vi "Vision Assistant2.vi"(0 "Image In":T1, 1 "Color Plane (Color Plane Extraction 1)":i32(ring)=2 items=["Red", "Green", "Blue", "Hue", "Saturation", "Luminance", "Value", "Intensity"], 2 "Range (Threshold 1)":cluster{"Lower value":sgl, "Upper value":sgl}={"Lower value"=199.0, "Upper value"=255.0}, 3 "Number of Erosion (Adv. Morphology 1)":i32=1, 4 "Square/Hexa (Square) (Adv. Morphology 1)":bool, 5 "Connectivity 4/8 (8) (Adv. Morphology 1)":bool=TRUE, 6 "Low Pass/High Pass (Low) (Adv. Morphology 1)":bool, 7 "error in":errorcluster) -> (20 "Image Out":T1, 21 "Number of Matches (Shape Matching 1)":i32, 22 "Shape Report (calibrated) (Shape Matching 1)":T2(array[cluster]) {"Score" format="%.2f"; "Centroid"."y" format="%.2f"; "Centroid"."x" format="%.2f"}, 23 "Centroid (Centroid 1)":cluster{"X Centroid":sgl, "Y Centroid":sgl} {"Y Centroid" format="%.2f"; "X Centroid" format="%.2f"}, 24 "Calibrated Centroid (Centroid 1)":cluster{"X Centroid":sgl, "Y Centroid":sgl} {"Y Centroid" format="%.2f"; "X Centroid" format="%.2f"}, 27 "error out":errorcluster)   [LabVIEW 2016]
uses:
  <vilib>/vision/Image Controls.llb/IMAQ Image.ctl
  Camera Global.vi
  <vilib>/vision/NI_Vision_Development_Module.lvlib
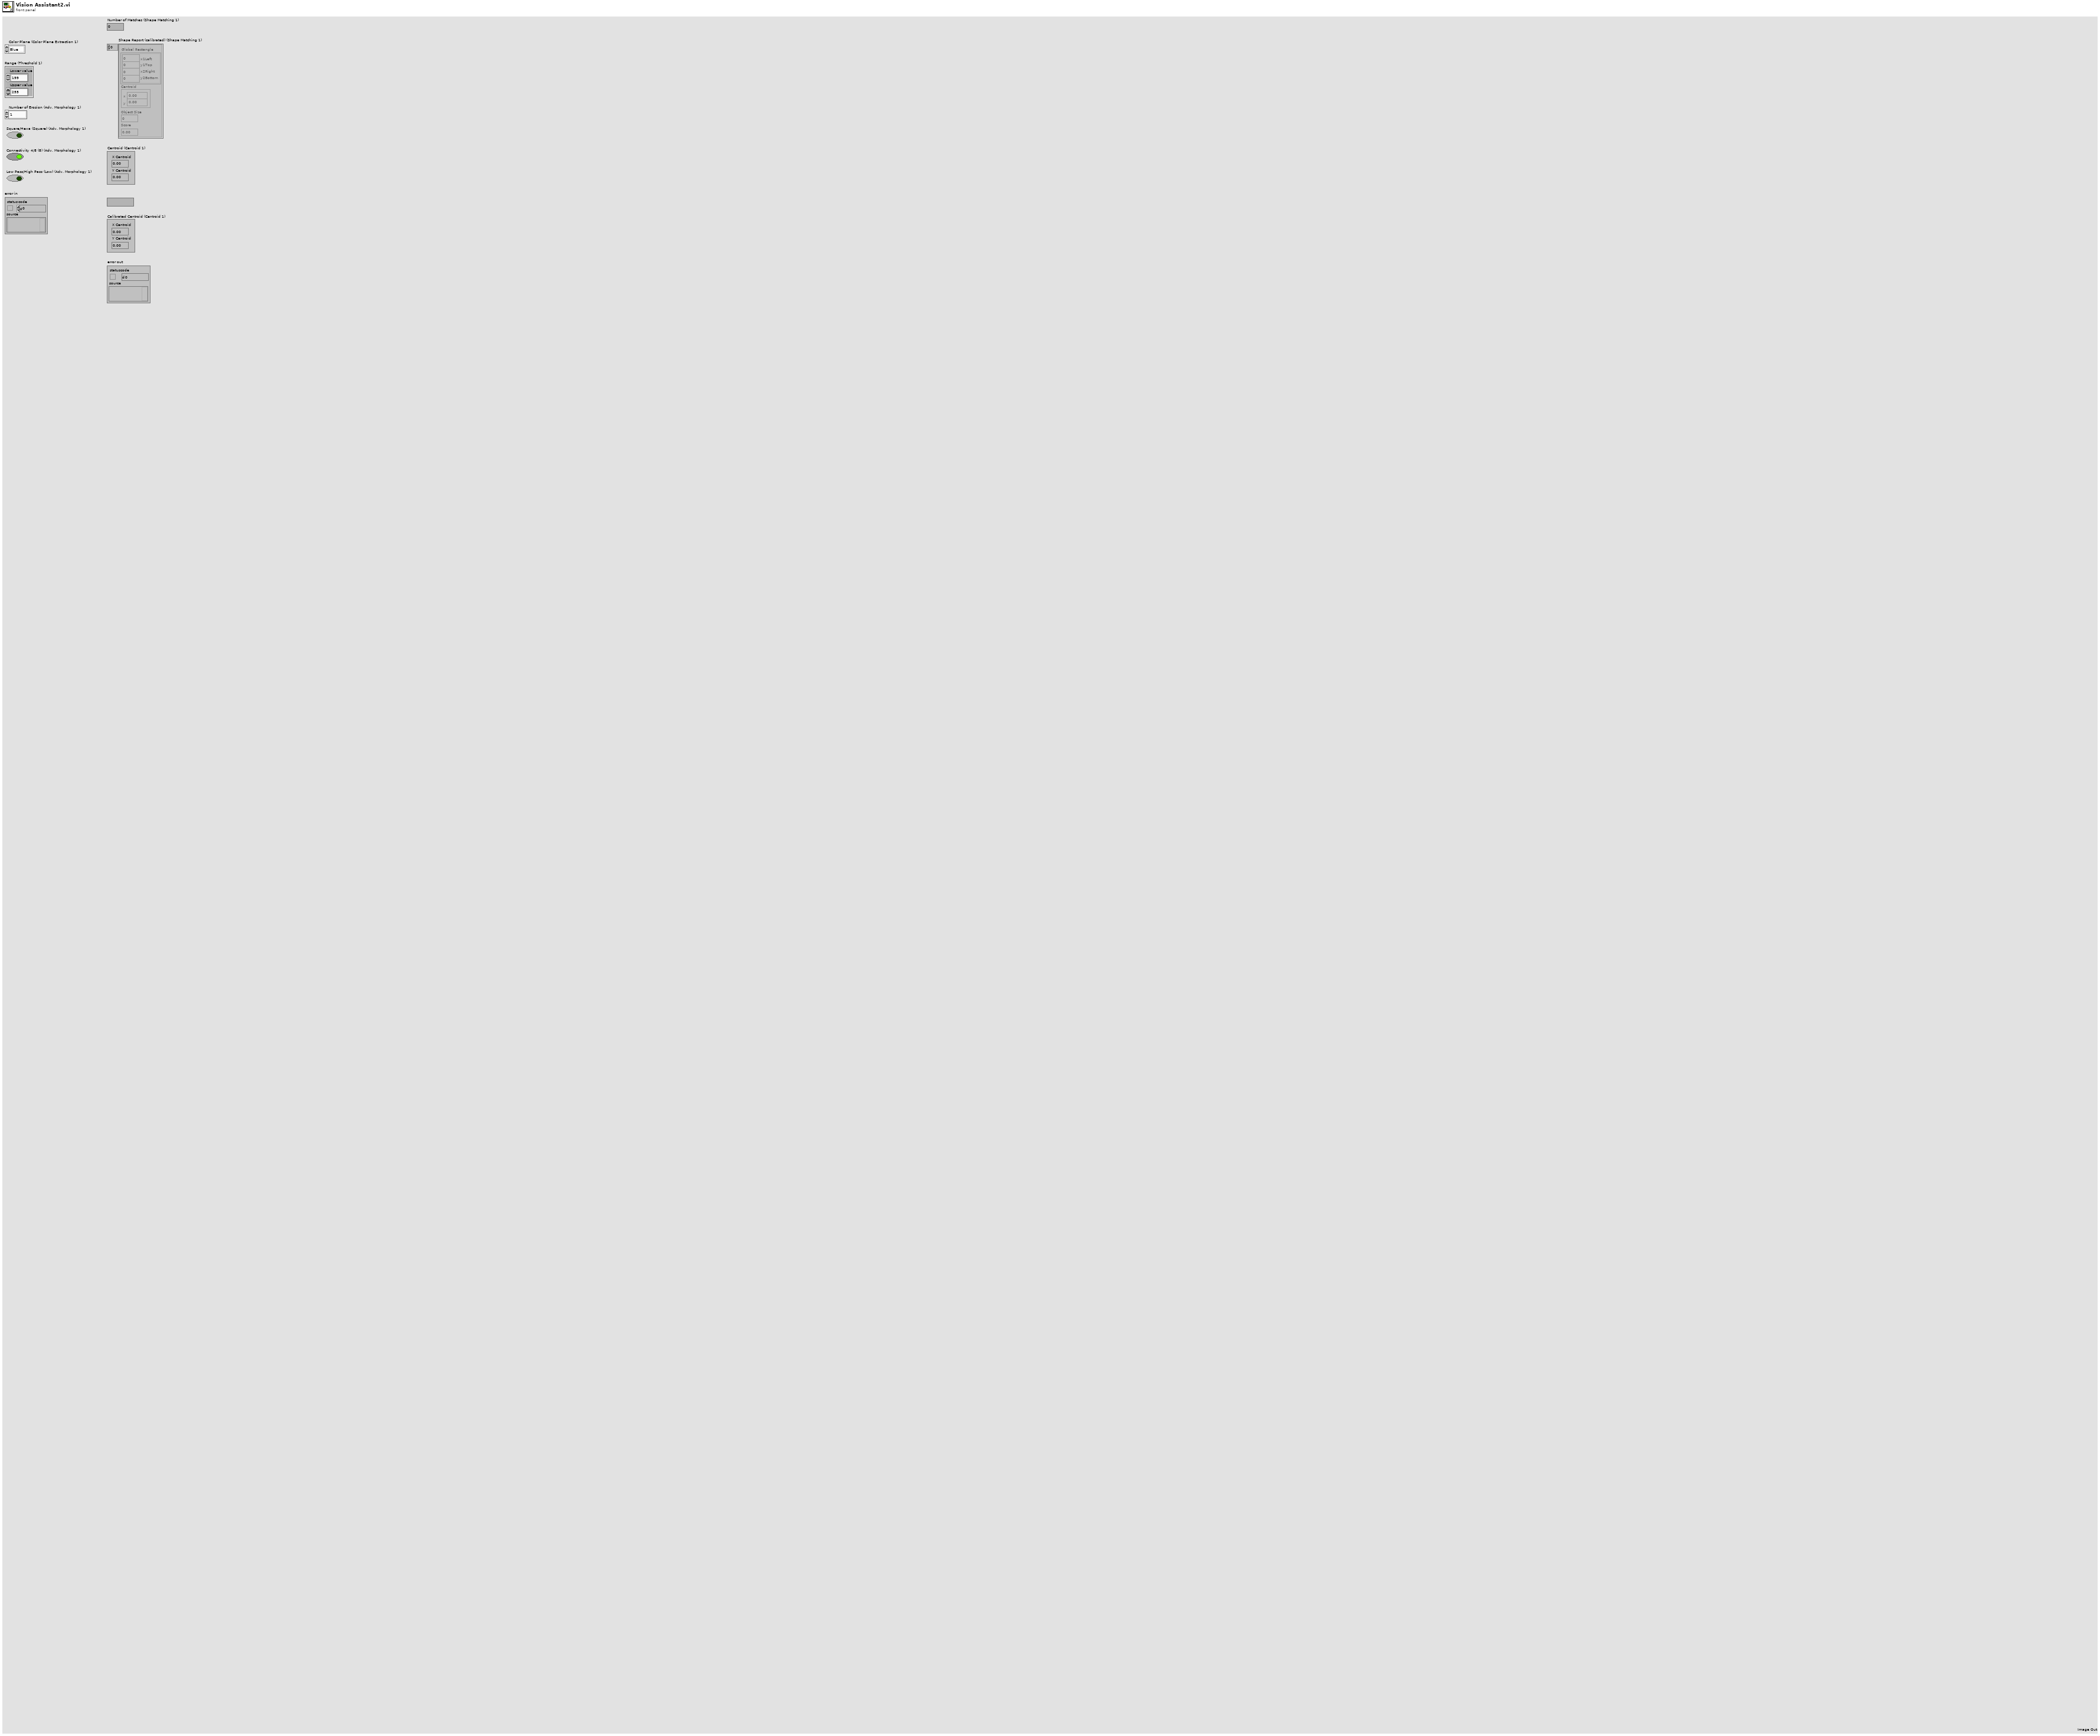
[diagram p1: front panel]
types:
  T1 = typedef "IMAQ Image.ctl" = refnum<image>
  T2 = cluster{"Global Rectangle":cluster{"x1Left":i32, "y1Top":i32, "x2Right":i32, "y2Bottom":i32}, "Centroid":cluster{"x":sgl, "y":sgl}, "Object Size":u32, "Score":dbl}[]
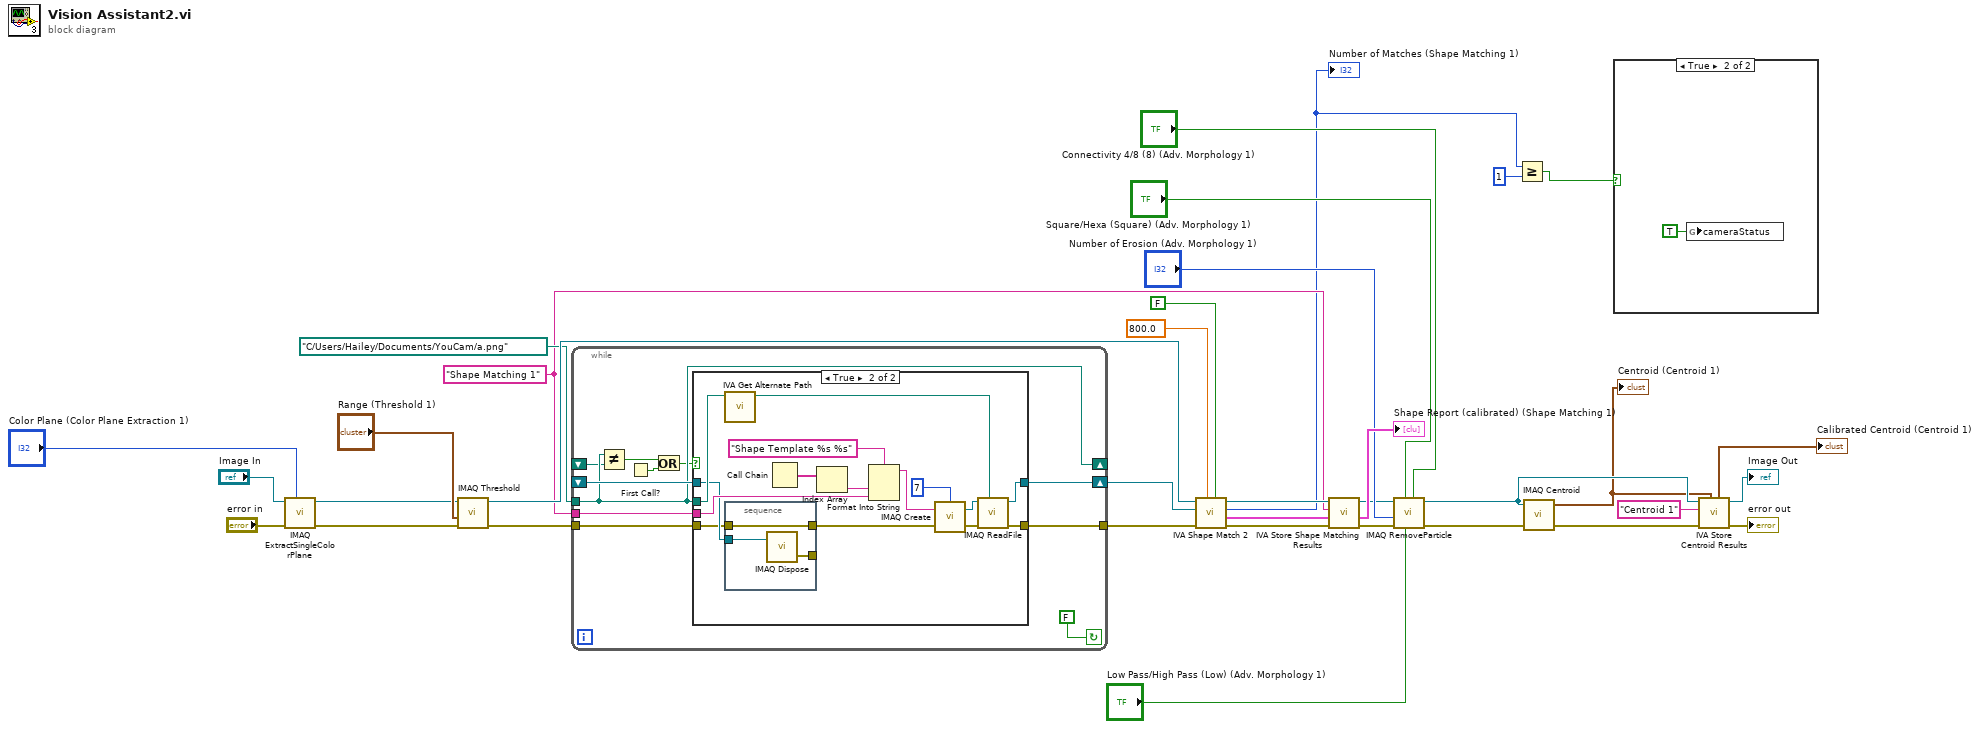
[diagram p0: block diagram]
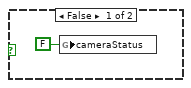
[diagram p2: hidden frame]
diagram:
  w17 = "Shape Matching 1" ("Step Name")
  n1 = call "IMAQ ExtractSingleColorPlane"("Color Plane"="Color Plane (Color Plane Extraction 1)", "error in (no error)"="error in", "Image Src"="Image In") -> ("error out"=w32:errorcluster, "Image Dst Out"=w30:T1)  [unwired: 1 in, 6 out]
  n2 = call "IMAQ Threshold"("error in (no error)"=w32, "Range"="Range (Threshold 1)", "Image Src"=w30) -> ("error out"=w29:errorcluster, "Image Dst Out"=w26:T1)  [unwired: 3 in, 4 out]
  n3 = while {
    shift-right: [w46] -> w18
    shift-left: _ -> [w45]
    tunnel: [w43] -> w19
    tunnel: w29 -> [w42]
    tunnel: path "C:/Users/Hailey/Documents/YouCam/a.png" ("Template Path") -> [w40]
    tunnel: w17 -> [w41]
    shift-right: [w40] -> _
    shift-left: _ -> [w39]
    stop <- FALSE continue-if-true
    n4 = Not Equal?(x=w40, y=w39) -> (x != y?=w37:bool)
    n5 = First Call?() -> (First Call?: T/F=w38:bool)
    n6 = Or(x=w37, y=w38) -> (x .or. y?=w36:bool)
    n7 = case shown="True" w36 {
      tunnel: [w48 w60] -> w46
      tunnel: w45 -> [w48 w51]
      tunnel: [w47 w58] -> w43
      tunnel: w42 -> [w47 w50]
      tunnel: w40 -> [_ w53]
      tunnel: w41 -> [_ w54]
      frame False {
      }
      frame True {
        n8 = call <vilib>:"IVA Get Alternate Path.vi"("Path In"=w53) -> ("Path Out"=w52:path)  [unwired: 10 out]
        n9 = stacked-sequence {
          tunnel: w51 -> [w66]
          tunnel: w50 -> [w65]
          tunnel: [w65] -> w49
          tunnel: [w64] -> _
          frame #0 {
            n10 = call "IMAQ Dispose"("Image"=w66) -> ("error out"=w64:errorcluster)  [unwired: 2 in, 3 out]
          }
        }
        n11 = Call Chain() -> (call chain=w56:string[])
        n12 = Index Array(array=w56) -> (element=w55:string)  [unwired: 1 in]
        n13 = Format Into String(format string="Shape Template %s %s" ("Image Name"), w55, w54) -> (resulting string=w63:string)  [unwired: 2 in, 1 out]
        n14 = call "IMAQ Create"("Border Size"=7, "Image Name"=w63, "error in (no error)"=w49) -> ("New Image"=w61:T1, "error out"=w59:errorcluster)  [unwired: 1 in, 1 out]
        n15 = call "IMAQ ReadFile"("File Path"=w52, "error in (no error)"=w59, "Image"=w61) -> ("error out"=w58:errorcluster, "Image Out"=w60:T1)  [unwired: 2 in, 5 out]
      }
    }
  }
  n16 = call <vilib>:"IVA Shape Match 2.vi"("Scale Invariance"=FALSE, "Minimal Score"=800.0, "error in (no error)"=w19, "Template"=w18, "Image Src"=w26) -> ("error out"=w25:errorcluster, "Shape Report"=w23:T2, "Number of Matches"=w3:i32, "Image Out"=w22:T1)  [unwired: 3 out]
  "Number of Matches (Shape Matching 1)" <- w3
  n17 = call <vilib>:"IVA Store Shape Matching Results.vi"("error in (no error)"=w25, "Shape Report"=w23, "Step Name"=w17, "Image in"=w22) -> ("error out"=w24:errorcluster, "Shape Report (calibrated)"=→"Shape Report (calibrated) (Shape Matching 1)":T2, "Image dup"=w12:T1)  [unwired: 5 out]
  n18 = call "IMAQ RemoveParticle"("Connectivity 4/8 (8)"="Connectivity 4/8 (8) (Adv. Morphology 1)", "Low Pass/High Pass (Low)"="Low Pass/High Pass (Low) (Adv. Morphology 1)", "Square/Hexa (Square)"="Square/Hexa (Square) (Adv. Morphology 1)", "error in (no error)"=w24, "Number of Erosion"="Number of Erosion (Adv. Morphology 1)", "Image Src"=w12) -> ("error out"=w11:errorcluster, "Image Dst Out"=w8:T1)  [unwired: 1 in, 3 out]
  n19 = Greater Or Equal?(x=w3, y=1) -> (x >= y?=w2:bool)
  n20 = call "IMAQ Centroid"("error in (no error)"=w11, "Image"=w8) -> ("error out"=w10:errorcluster, "Centroid"=w5:cluster{"X Centroid":sgl, "Y Centroid":sgl})  [unwired: 1 in, 1 out]
  "Centroid (Centroid 1)" <- w5
  n21 = case shown="True" w2 {
    frame False {
      n22 = global write "Camera Global.vi" "cameraStatus"(FALSE ("cameraStatus")) -> ()
    }
    frame True {
      n23 = global write "Camera Global.vi" "cameraStatus"(TRUE ("cameraStatus")) -> ()
    }
  }
  n24 = call <vilib>:"IVA Store Centroid Results.vi"("Centroid in"=w5, "error in (no error)"=w10, "Step Name"="Centroid 1", "Image in"=w8) -> ("error out"=→"error out":errorcluster, "Image dup"=→"Image Out":T1, "Calibrated Centroid"=→"Calibrated Centroid (Centroid 1)":cluster{"X":sgl, "Y":sgl})  [unwired: 5 out]
